vi "Move Cell.vi"(8 "error in (no error)":errorcluster, 9 "Up/Down":bool=TRUE, 10 "Cell index":i32, 11 "Schedule in":refnum<class "Schedule.lvclass">) -> (0 "error out":errorcluster, 2 "New index":i32=-1, 3 "Schedule out":refnum<class "Schedule.lvclass">)   [LabVIEW 2020, in "Run Utilities.lvlib" / "Schedule.lvclass"]
doc: "Move specified cell <b>Up</b>(<b>True</b>) or <b>Down</b> (<b>False</b>) in the schedule.\nIf any of the indices for the move is invalid the VI will ignore the move operation and the schedule stays unchanged"
uses:
  Schedule.lvclass
  Schedule.lvclass/Schedule.ctl
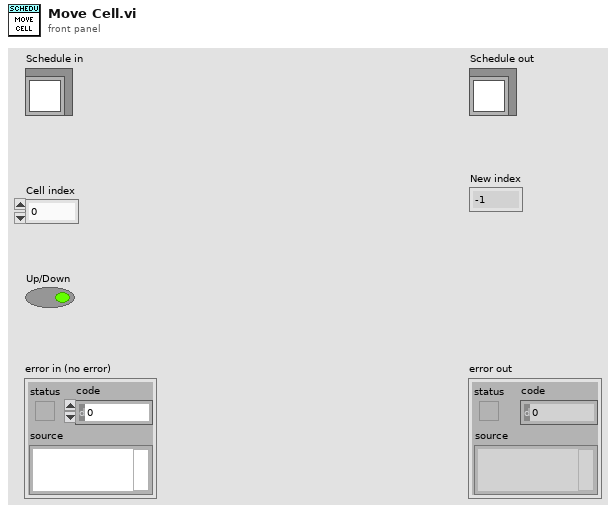
[diagram p1: front panel]
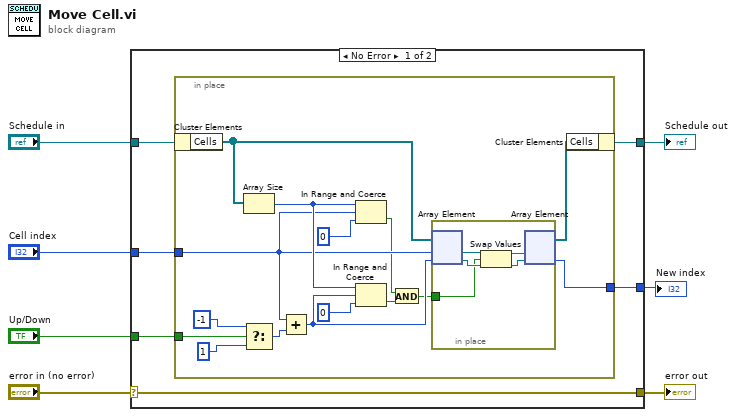
[diagram p0: block diagram]
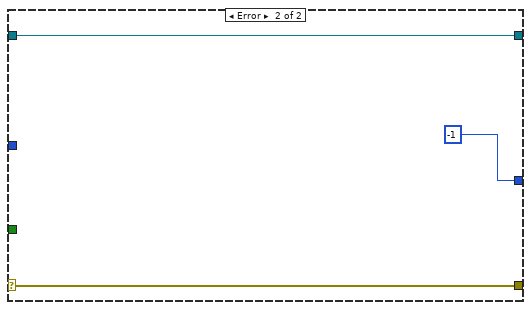
[diagram p2: hidden frame]
diagram:
  n1 = case shown="No Error" "error in (no error)" {
    selector: "error in (no error)" -> [w13 w36]
    tunnel: [w13 w36] -> w6
    tunnel: [w11 w35] -> w4
    tunnel: "Schedule in" -> [w12 w35]
    tunnel: "Cell index" -> [w10 _]
    tunnel: "Up/Down" -> [w9 _]
    tunnel: [w8 -1] -> w1
    frame No Error {
      n2 = in-place {
        in-place-border: w10 -> [w20]
        in-place-border: w9 -> [w25]
        in-place-border: [w14] -> w8
        n3 = in-place-cluster #1(w12) -> ("Cells"=w21:refnum<class "Schedule Cell.lvclass">[])
        n4 = Array Size(array=w21) -> (size(s)=w27:i32)
        n5 = Select(t=-1 ("Cell index"), s=w25, f=1 ("Cell index")) -> (s? t:f=w24:i32)
        n6 = Add(x=w20, y=w24) -> (x+y=w28:i32)
        n7 = In Range and Coerce(upper limit=w27, x=w20, lower limit=0) -> (In Range?=w16:bool)  [unwired: 1 out]
        n8 = In Range and Coerce(upper limit=w27, x=w28, lower limit=0) -> (In Range?=w17:bool)  [unwired: 1 out]
        n9 = And(x=w16, y=w17) -> (x .and. y?=w15:bool)
        n10 = in-place {
          in-place-border: w15 -> [w29]
          n11 = in-place-array #2(w21, w20, w28) -> (w33:refnum<class "Schedule Cell.lvclass">, w32:refnum<class "Schedule Cell.lvclass">)
          n12 = Swap Values(12:w33, 13:w29, 14:w32) -> (1:w31:refnum<class "Schedule Cell.lvclass">, 3:w30:refnum<class "Schedule Cell.lvclass">)
          n13 = in-place-array #2(w31, w30) -> (w26:refnum<class "Schedule Cell.lvclass">[], w14:i32)  [unwired: 1 out]
        }
        n14 = in-place-cluster #1("Cells"=w26) -> (w11:refnum<class "Schedule.lvclass">)
      }
    }
    frame Error {
    }
  }
  "error out" <- w6
  "Schedule out" <- w4
  "New index" <- w1
